vi "Initialize Sequences.vi"(8 "error in (no error)":errorcluster, 9 "data allocations":T1, 11 "Customize:Properties:Lines":T4[](array[typedef])) -> (0 "error out":errorcluster, 3 "Array":refnum<class "Sequence.lvclass">[](array[class]))   [LabVIEW 2015, in "Sequencer Module runtime.lvclass"]
uses:
  Sequencer Module runtime.lvclass
  classes/Sequence/Execution/Sequence.lvclass
  configuration/Line.ctl
  classes/Sequence/Config/Sequence Config.lvclass
  <vilib>/NI/Tag Bus Module Framework/channel/data tables.ctl
  <vilib>/NI/Tag Bus/dictionary/data dictionary.lvclass
  <vilib>/NI/Tag Bus/dictionary table pair.ctl
  <vilib>/NI/Tag Bus/table/data table.ctl
  configuration/Sequencer Module configuration.lvclass
  <vilib>/NI/Tag Bus/table/data table.lvlib
  <vilib>/NI/Tag Bus/tag bus.lvlib
  <vilib>/NI/Tag Bus Module Framework/channel/TBM channel.lvclass
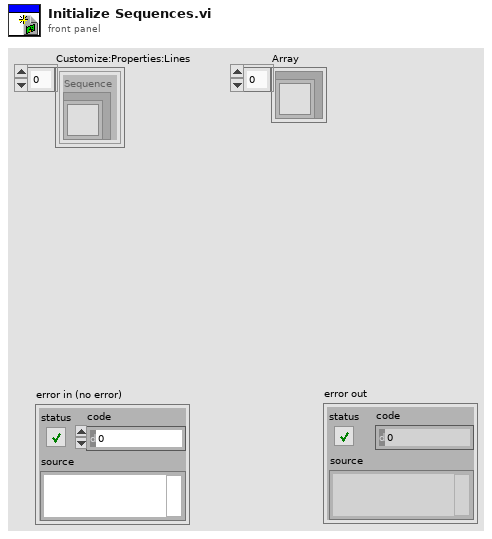
[diagram p1: front panel]
types:
  T1 = typedef "TBM channel.lvclass/data tables.ctl" = cluster{"input data":T2, "processing parameter":T2, "processing result":T2, "output data":T2}
  T2 = typedef "tag bus.lvlib/dictionary table pair.ctl" = cluster{"data dictionary":refnum<class "data dictionary.lvclass">, "data table":T3}
  T3 = typedef "tag bus.lvlib/data table.lvlib/data table.ctl" = cluster{"Double":dbl[], "Single":sgl[], "I64":i64[], "I32":i32[], "I16":i16[], "I8":i8[], "U64":u64[], "U32":u32[], "U16":u16[], "U8":u8[], "Boolean":bool[], "String":string[], "Array of Double":cluster{"DBL Array":dbl[]}[], "Array of Single":cluster{"SGL Array":sgl[]}[], "Array of I64":cluster{"I64 Array":i64[]}[], "Array of I32":cluster{"I32 Array":i32[]}[], "Array of I16":cluster{"I16 Array":i16[]}[], "Array of I8":cluster{"I8 Array":i8[]}[], "Array of U64":cluster{"U64 Array":u64[]}[], "Array of U32":cluster{"U32 Array":u32[]}[], "Array of U16":cluster{"U16 Array":u16[]}[], "Array of U8":cluster{"U8 Array":u8[]}[], "Array of Boolean":cluster{"Boolean Array":bool[]}[], "Array of String":cluster{"String Array":string[]}[]}
  T4 = typedef "Sequencer Module configuration.lvclass/Line.ctl" = cluster{"Sequence":refnum<class "Sequence Config.lvclass">}
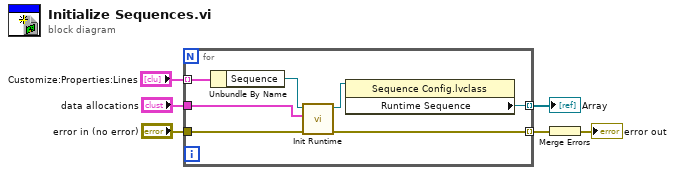
[diagram p0: block diagram]
diagram:
  n1 = for {
    tunnel: "Customize:Properties:Lines" -> [w13] mode=indexing
    tunnel: [w8] -> w6 mode=indexing
    tunnel: "data allocations" -> [w11]
    tunnel: "error in (no error)" -> [w10]
    tunnel: [w7] -> w2 mode=indexing
    n2 = Unbundle By Name(w13) -> ("Sequence"=w12:refnum<class "Sequence Config.lvclass">)
    n3 = call-dynamic "Init Runtime.vi"("error in (no error)"=w10, "data allocations"=w11, "Sequence Config in"=w12) -> ("error out"=w7:errorcluster, "Sequence Config out"=w9:refnum<class "Sequence Config.lvclass">)  [unwired: 7 in]
    n4 = property class="Sequence Config.lvclass"(reference=w9) -> ("Runtime Sequence"=w8:refnum<class "Sequence.lvclass">)  [unwired: 1 in, 2 out]
  }
  "Array" <- w6
  n5 = Merge Errors(w2) -> (→"error out":errorcluster)
